vi "Create Methods.vi"(8 "error in (no error)":errorcluster, 11 "protoFile ref in":u64) -> (0 "error out":errorcluster, 3 "Method Parameters":T1[](array[typedef]))   [LabVIEW 2019, in "gRPC Template Creation Utility.lvlib"]
uses:
  gRPC Template Creation Utility.lvlib
  TypeDefs/RPC Method Parameters.ctl
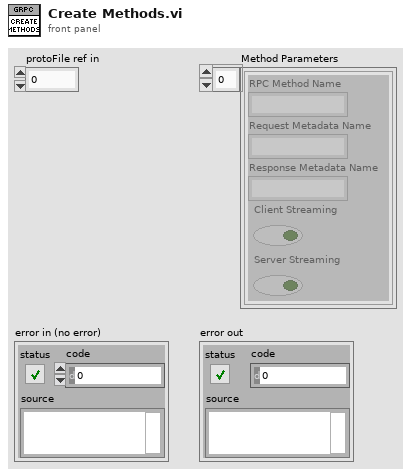
[diagram p1: front panel]
types:
  T1 = typedef "gRPC Template Creation Utility.lvlib/RPC Method Parameters.ctl" = cluster{"RPC Method Name":string, "Request Metadata Name":string, "Response Metadata Name":string, "Client Streaming":bool, "Server Streaming":bool}
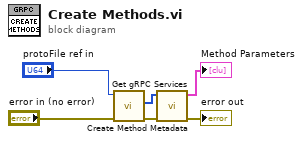
[diagram p0: block diagram]
diagram:
  n1 = call "Get gRPC Services.vi"("error in (no error)"="error in (no error)", "protoFile ref in"="protoFile ref in") -> ("error out"=w6:errorcluster, "services"=w1:u64[])  [unwired: 7 in, 1 out]
  n2 = call "Create Method Metadata.vi"("error in (no error)"=w6, "services"=w1) -> ("error out"=→"error out":errorcluster, "Method Parameters"=→"Method Parameters":T1[])  [unwired: 8 in]
